vi "Get goto instructions.vi"(8 "error in (no error)":errorcluster, 11 "Motor in":refnum<class "Motor.lvclass">) -> (0 "error out":errorcluster, 1 "name":string, 2 "goto instructions":string[](array[string]), 3 "Motor out":refnum<class "Motor.lvclass">)   [LabVIEW 2018, in "Motor.lvclass"]
uses:
  Motor.lvclass
  Motor.lvclass/Motor.ctl
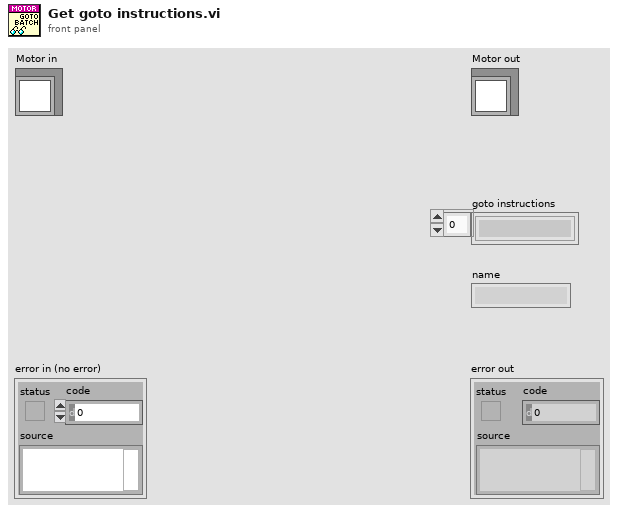
[diagram p1: front panel]
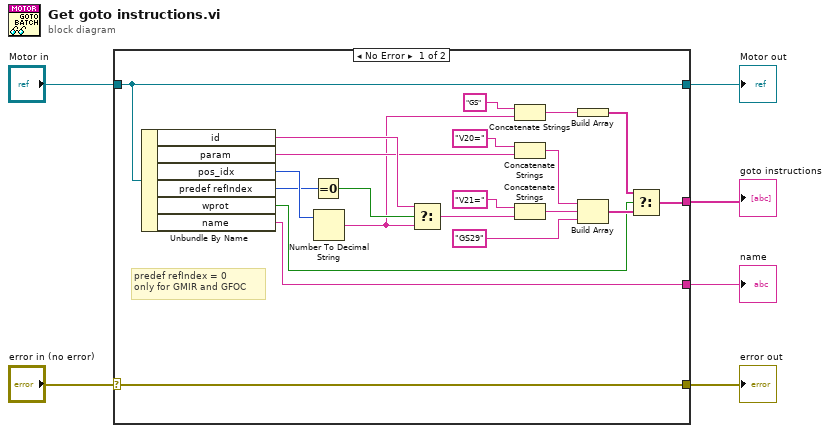
[diagram p0: block diagram]
diagram:
  n1 = case shown="No Error" "error in (no error)" {
    selector: "error in (no error)" -> [w27 w28]
    tunnel: [w27 w28] -> w5
    tunnel: [w26 w29] -> w3
    tunnel: "Motor in" -> [w26 w29]
    tunnel: [w14 _] -> w2
    tunnel: [w7 _] -> w1
    frame No Error {
      # "predef refIndex = 0\nonly for GMIR and GFOC"
      n2 = Unbundle By Name(w26) -> ("id"=w18:string, "param"=w17:string, "pos_idx"=w21:i32, "predef refIndex"=w20:i32, "wprot"=w8:bool, "name"=w7:string)
      n3 = Equal To 0?(x=w20) -> (x = 0?=w19:bool)
      n4 = Number To Decimal String(number=w21) -> (decimal integer string=w11:string)  [unwired: 1 in]
      n5 = Select(t=w18, s=w19, f=w11) -> (s? t:f=w16:string)
      n6 = Concatenate Strings("GS" ("string"), w11) -> (w10:string)
      n7 = Concatenate Strings("V20=" ("string"), w17) -> (w13:string)
      n8 = Concatenate Strings("V21=" ("string"), w16) -> (w23:string)
      n9 = Build Array(w10) -> (w9:string[])
      n10 = Build Array(w13, w23, "GS29" ("string")) -> (w15:string[])
      n11 = Select(t=w9, s=w8, f=w15) -> (s? t:f=w14:string[])
    }
    frame Error {
    }
  }
  "error out" <- w5
  "Motor out" <- w3
  "goto instructions" <- w2
  "name" <- w1
